vi "PH_PP_CurrentMeas.PC _PU Status.vi"(0 "i ref in":refnum<vi>, 2 "serviceName":string, 3 "Status":T1 items=["no info", "off/false/out", "on/true/in", "Failure", "Alarm", "Status 1", "Status 2", "Status 3"], 4 "no link":bool, 5 "error in (no error)":errorcluster) -> (14 "i ref out":refnum<vi>, 19 "error out":errorcluster)   [LabVIEW 2014, in "PH_PP_CurrentMeas.lvlib"]
uses:
  PH_PP_CurrentMeas.lvlib
  PH_Basics/PH_StatusHandler/PH_StatusHandler.Status.ctl
  PH_Basics/PH_StatusHandler/PH_StatusHandler.lvlib
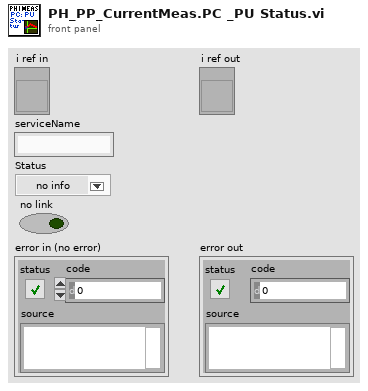
[diagram p1: front panel]
types:
  T1 = typedef "PH_StatusHandler.lvlib/PH_StatusHandler.Status.ctl" = i16
  T2 = typedef "PH_PP_CurrentMeas.lvlib/PH_PP_CurrentMeas.i attribute.ctl" = cluster{"Status":cluster{"GUI Ref Hardware Feedback":refnum<vi>, "Tab Control":refnum<vi>}, "PU 1":cluster{"Instance":string, "Status":T1, "Ref Status ":refnum<vi>, "Data":waveform(dbl)[], "Ref Data":refnum<vi>}, "PU 2":cluster{"Instance":string, "Status":T1, "Ref Status ":refnum<vi>, "Data":waveform(dbl)[], "Ref Data":refnum<vi>}, "PU 3":cluster{"Instance":string, "Status":T1, "Ref Status ":refnum<vi>, "Data":waveform(dbl)[], "Ref Data":refnum<vi>}, "PU 4":cluster{"Instance":string, "Status":T1, "Ref Status ":refnum<vi>, "Data":waveform(dbl)[], "Ref Data":refnum<vi>}, "PU 5":cluster{"Instance":string, "Status":T1, "Ref Status ":refnum<vi>, "Data":waveform(dbl)[], "Ref Data":refnum<vi>}, "FR":cluster{"Instance":string, "Status":T1, "Ref Status ":refnum<vi>, "Data":waveform(dbl)[], "Ref Data":refnum<vi>}, "PA - 19mm 1":cluster{"Instance":string, "Status":T1, "Ref Status ":refnum<vi>}, "PA - 19mm 2":cluster{"Instance":string, "Status":T1, "Ref Status ":refnum<vi>, "no link":bool}, "PA - 45mm":cluster{"Instance":string, "Status":T1, "Ref Status ":refnum<vi>, "no link":bool}, "PA Data":cluster{"Data":waveform(dbl)[], "Ref":refnum<vi>}, "Sequencer":cluster{"Instance":string, "SM State Ref":refnum<vi>}, "Tasks":cluster{"Port":u16, "connection ID":refnum<k5>, "Status":T1, "Ref":refnum<vi>, "Ref Bar":refnum<vi>, "Feedback":cluster{"Received Data Sets":T3[], "Driver Error":errorcluster, "Connection not established":bool, "Error unpacking the data":bool, "No Task defined":bool, "Not triggered yet":bool}, "Data":waveform(dbl)[], "Ref Teststart Task":refnum<vi>}[], "in use":cluster{"MA DP":bool, "FR and PA":bool}, "DAQ Server":string}
  T3 = typedef "PH_PP_CurrentMeas.lvlib/PH_PP_CurrentMeas.CommandCluster.ctl" = cluster{"Command":string, "Data":string, "error out":errorcluster}
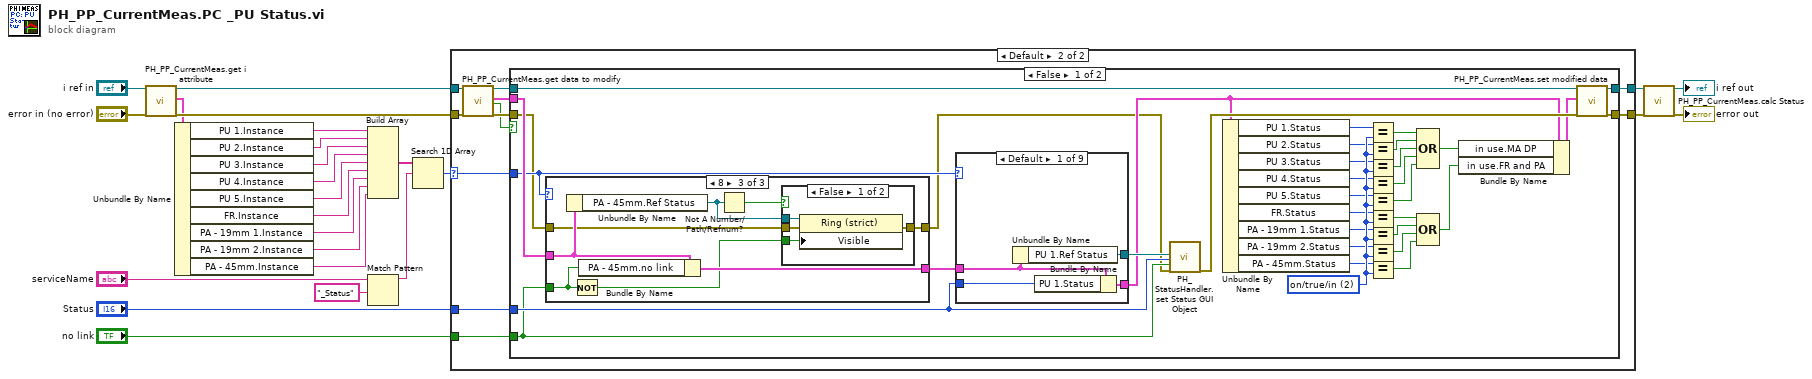
[diagram p0: block diagram]
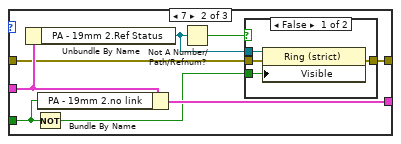
[diagram p4: hidden frame]
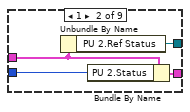
[diagram p7: hidden frame]
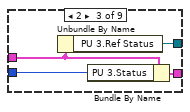
[diagram p8: hidden frame]
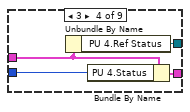
[diagram p9: hidden frame]
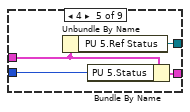
[diagram p10: hidden frame]
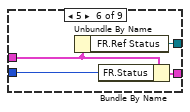
[diagram p11: hidden frame]
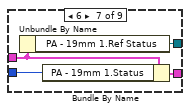
[diagram p12: hidden frame]
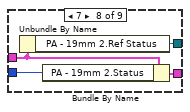
[diagram p13: hidden frame]
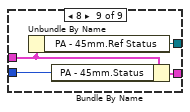
[diagram p14: hidden frame]
diagram:
  n1 = call "PH_PP_CurrentMeas.get i attribute.vi"("i ref in"="i ref in", "error in (no error)"="error in (no error)") -> ("i ref out"=w19:refnum<vi>, "i attribute"=w3:T2, "error out"=w15:errorcluster)  [unwired: 15 in]
  n2 = Unbundle By Name(w3) -> ("PU 1.Instance"=w4:string, "PU 2.Instance"=w5:string, "PU 3.Instance"=w6:string, "PU 4.Instance"=w7:string, "PU 5.Instance"=w8:string, "FR.Instance"=w9:string, "PA - 19mm 1.Instance"=w10:string, "PA - 19mm 2.Instance"=w11:string, "PA - 45mm.Instance"=w12:string)
  n3 = Build Array(w4, w5, w6, w7, w8, w9, w10, w11, w12) -> (w16:string[])
  n4 = Match Pattern(string="serviceName", regular expression="_Status") -> (before substring=w17:string)  [unwired: 1 in, 3 out]
  n5 = Search 1D Array(1D array=w16, element=w17) -> (index of element=w21:i32)  [unwired: 1 in]
  n6 = case shown="Default" w21 {
    selector: w21 -> [_ w28]
    tunnel: w15 -> [w26 w38]
    tunnel: [w26 w36] -> w18
    tunnel: w19 -> [w27 w35]
    tunnel: [w27 w33] -> w24
    tunnel: "Status" -> [_ w30]
    tunnel: "no link" -> [_ w29]
    frame -1 {
    }
    frame Default {
      n7 = call "PH_PP_CurrentMeas.get data to modify.vi"("i ref in"=w35, "error in (no error)"=w38) -> ("i ref out"=w34:refnum<vi>, "i attribute"=w31:T2, "timed out"=w32:bool, "error out"=w37:errorcluster)  [unwired: 14 in]
      n8 = case shown="False" w32 {
        tunnel: w37 -> [w40 w138]
        tunnel: [w70 w138] -> w36
        tunnel: w34 -> [w73 w139]
        tunnel: [w72 w139] -> w33
        tunnel: w31 -> [w45 _]
        tunnel: w30 -> [w43 _]
        tunnel: w29 -> [w42 _]
        tunnel: w28 -> [w41 _]
        frame False {
          w59 = T1 2 items=["no info", "off/false/out", "on/true/in", "Failure", "Alarm", "Status 1", "Status 2", "Status 3"] ("y")
          n9 = case shown="8" w41 {
            tunnel: [w75 w83 w96] -> w44
            tunnel: w45 -> [w75 w82 w95]
            tunnel: w42 -> [_ w81 w94]
            tunnel: w40 -> [w74 w77 w90]
            tunnel: [w74 w76 w89] -> w39
            frame Default {
            }
            frame 7 {
              n10 = Unbundle By Name(w82) -> ("PA - 19mm 2.Ref Status"=w78:refnum<vi>)
              n11 = Not(x=w81) -> (.not. x?=w80:bool)
              n12 = Bundle By Name(cluster=w82, "PA - 19mm 2.no link"=w81) -> (w83:T2)
              n13 = Not A Number/Path/Refnum?(number/path/refnum=w78) -> (NaN/Path/Refnum?=w79:bool)
              n14 = case shown="False" w79 {
                tunnel: w78 -> [w87 _]
                tunnel: w80 -> [w86 _]
                tunnel: w77 -> [w85 w88]
                tunnel: [w84 w88] -> w76
                frame False {
                  n15 = property class="Ring (strict)"(reference=w87, error in=w85, "Visible"=w86) -> (error out=w84:errorcluster)  [unwired: 1 out]
                }
                frame True {
                }
              }
            }
            frame 8 {
              n16 = Unbundle By Name(w95) -> ("PA - 45mm.Ref Status"=w91:refnum<vi>)
              n17 = Not(x=w94) -> (.not. x?=w93:bool)
              n18 = Bundle By Name(cluster=w95, "PA - 45mm.no link"=w94) -> (w96:T2)
              n19 = Not A Number/Path/Refnum?(number/path/refnum=w91) -> (NaN/Path/Refnum?=w92:bool)
              n20 = case shown="False" w92 {
                tunnel: w91 -> [w100 _]
                tunnel: w93 -> [w99 _]
                tunnel: w90 -> [w98 w101]
                tunnel: [w97 w101] -> w89
                frame False {
                  n21 = property class="Ring (strict)"(reference=w100, error in=w98, "Visible"=w99) -> (error out=w97:errorcluster)  [unwired: 1 out]
                }
                frame True {
                }
              }
            }
          }
          n22 = case shown="Default" w41 {
            tunnel: [w105 w109 w113 w117 w121 w125 w129 w133 w137] -> w46
            tunnel: w44 -> [w104 w108 w112 w116 w120 w124 w128 w132 w136]
            tunnel: [w103 w107 w111 w115 w119 w123 w127 w131 w135] -> w71
            tunnel: w43 -> [w102 w106 w110 w114 w118 w122 w126 w130 w134]
            frame Default {
              n23 = Unbundle By Name(w104) -> ("PU 1.Ref Status"=w103:refnum<vi>)
              n24 = Bundle By Name(cluster=w104, "PU 1.Status"=w102) -> (w105:T2)
            }
            frame 1 {
              n25 = Unbundle By Name(w108) -> ("PU 2.Ref Status"=w107:refnum<vi>)
              n26 = Bundle By Name(cluster=w108, "PU 2.Status"=w106) -> (w109:T2)
            }
            frame 2 {
              n27 = Unbundle By Name(w112) -> ("PU 3.Ref Status"=w111:refnum<vi>)
              n28 = Bundle By Name(cluster=w112, "PU 3.Status"=w110) -> (w113:T2)
            }
            frame 3 {
              n29 = Unbundle By Name(w116) -> ("PU 4.Ref Status"=w115:refnum<vi>)
              n30 = Bundle By Name(cluster=w116, "PU 4.Status"=w114) -> (w117:T2)
            }
            frame 4 {
              n31 = Unbundle By Name(w120) -> ("PU 5.Ref Status"=w119:refnum<vi>)
              n32 = Bundle By Name(cluster=w120, "PU 5.Status"=w118) -> (w121:T2)
            }
            frame 5 {
              n33 = Unbundle By Name(w124) -> ("FR.Ref Status"=w123:refnum<vi>)
              n34 = Bundle By Name(cluster=w124, "FR.Status"=w122) -> (w125:T2)
            }
            frame 6 {
              n35 = Unbundle By Name(w128) -> ("PA - 19mm 1.Ref Status"=w127:refnum<vi>)
              n36 = Bundle By Name(cluster=w128, "PA - 19mm 1.Status"=w126) -> (w129:T2)
            }
            frame 7 {
              n37 = Unbundle By Name(w132) -> ("PA - 19mm 2.Ref Status"=w131:refnum<vi>)
              n38 = Bundle By Name(cluster=w132, "PA - 19mm 2.Status"=w130) -> (w133:T2)
            }
            frame 8 {
              n39 = Unbundle By Name(w136) -> ("PA - 45mm.Ref Status"=w135:refnum<vi>)
              n40 = Bundle By Name(cluster=w136, "PA - 45mm.Status"=w134) -> (w137:T2)
            }
          }
          n41 = call "PH_StatusHandler.set Status GUI Object.vi"("PH Status Ref"=w71, "Value"=w43, "Blinking (false)"=w42, "error in (no error)"=w39) -> ("error out"=w69:errorcluster)  [unwired: 15 in]
          n42 = Unbundle By Name(w46) -> ("PU 1.Status"=w50:T1, "PU 2.Status"=w51:T1, "PU 3.Status"=w52:T1, "PU 4.Status"=w53:T1, "PU 5.Status"=w54:T1, "FR.Status"=w55:T1, "PA - 19mm 1.Status"=w56:T1, "PA - 19mm 2.Status"=w57:T1, "PA - 45mm.Status"=w58:T1)
          n43 = Equal?(x=w50, y=w59) -> (x = y?=w60:bool)
          n44 = Equal?(x=w51, y=w59) -> (x = y?=w61:bool)
          n45 = Equal?(x=w52, y=w59) -> (x = y?=w62:bool)
          n46 = Equal?(x=w53, y=w59) -> (x = y?=w63:bool)
          n47 = Equal?(x=w54, y=w59) -> (x = y?=w64:bool)
          n48 = Equal?(x=w55, y=w59) -> (x = y?=w65:bool)
          n49 = Equal?(x=w56, y=w59) -> (x = y?=w66:bool)
          n50 = Equal?(x=w57, y=w59) -> (x = y?=w67:bool)
          n51 = Equal?(x=w58, y=w59) -> (x = y?=w68:bool)
          n52 = Compound Arithmetic op=OR(w60, w61, w62, w63, w64) -> (w49:bool)
          n53 = Compound Arithmetic op=OR(w65, w66, w67, w68) -> (w48:bool)
          n54 = Bundle By Name(cluster=w46, "in use.MA DP"=w49, "in use.FR and PA"=w48) -> (w47:T2)
          n55 = call "PH_PP_CurrentMeas.set modified data.vi"("i ref in"=w73, "i attribute"=w47, "error in (no error)"=w69) -> ("i ref out"=w72:refnum<vi>, "error out"=w70:errorcluster)  [unwired: 15 in]
        }
        frame True {
        }
      }
    }
  }
  n56 = call "PH_PP_CurrentMeas.calc Status.vi"("i ref in"=w24, "error in (no error)"=w18) -> ("i ref out"=→"i ref out":refnum<vi>, "error out"=→"error out":errorcluster)  [unwired: 16 in]
